vi "Move.vi"(6 "Cost":i32, 8 "Hallway Index":i32, 9 "Column Index":i32, 10 "Column":string, 11 "Data In":T1) -> (3 "Data Out":T1)   [LabVIEW 2020]
uses:
  Data.ctl
  <userlib>/_OpenG.lib/array/array.llb/Index 1D Array Elements (String)__ogtk.vi
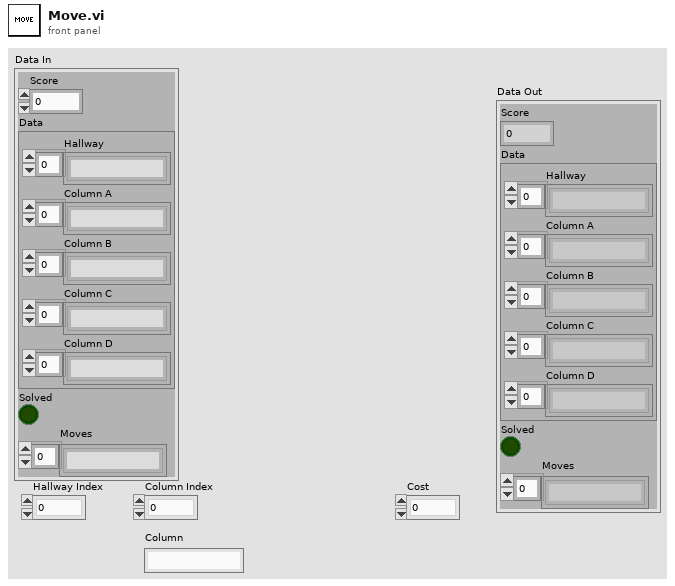
[diagram p1: front panel]
types:
  T1 = typedef "Data.ctl" = cluster{"Score":i64, "Data":cluster{"Hallway":string[], "Column A":string[], "Column B":string[], "Column C":string[], "Column D":string[]}, "Solved":bool, "Moves":string[]}
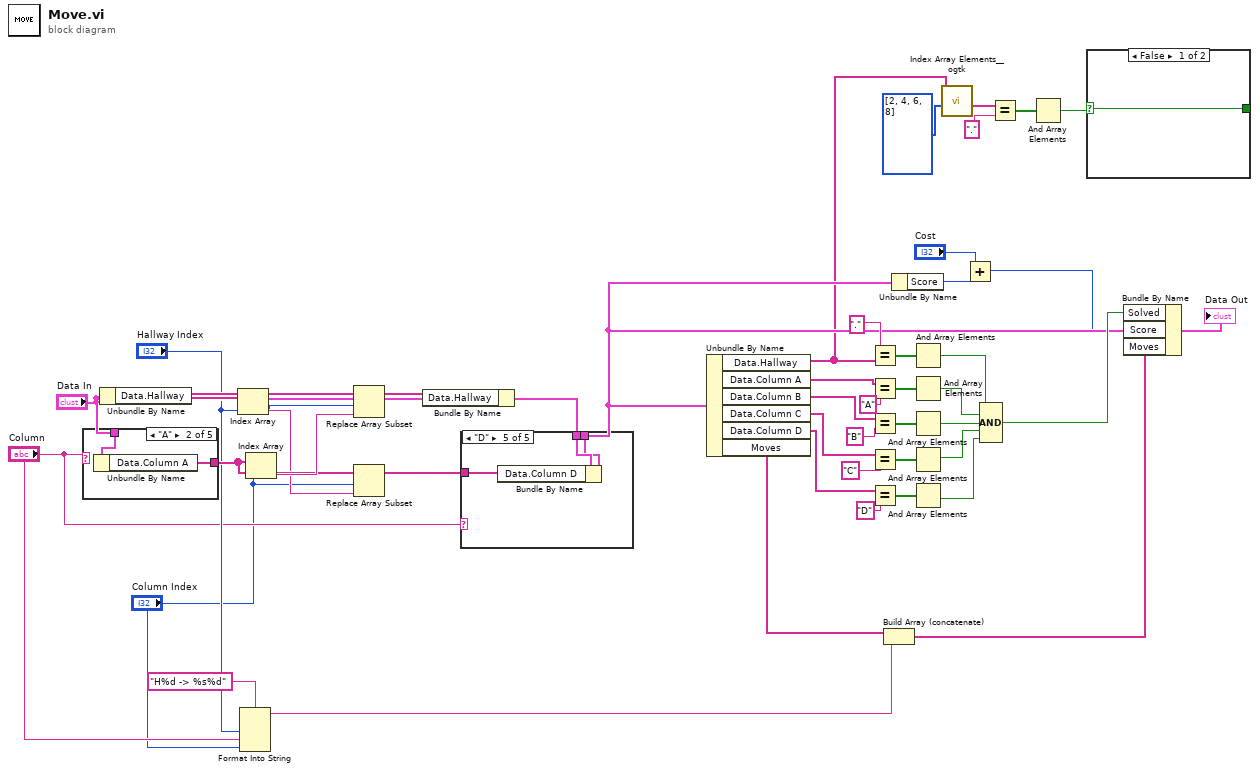
[diagram p0: block diagram]
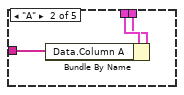
[diagram p4: hidden frame]
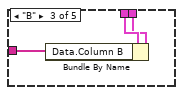
[diagram p5: hidden frame]
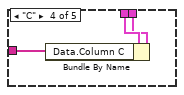
[diagram p6: hidden frame]
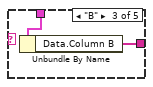
[diagram p8: hidden frame]
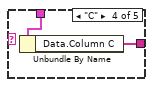
[diagram p9: hidden frame]
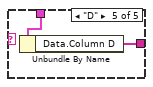
[diagram p10: hidden frame]
diagram:
  n1 = case shown="\"A\"" "Column" {
    tunnel: "Data In" -> [_ w48 w50 w52 w54]
    tunnel: [_ w47 w49 w51 w53] -> w44
    frame Default {
    }
    frame "A" {
      n2 = Unbundle By Name(w48) -> ("Data.Column A"=w47:string[])
    }
    frame "B" {
      n3 = Unbundle By Name(w50) -> ("Data.Column B"=w49:string[])
    }
    frame "C" {
      n4 = Unbundle By Name(w52) -> ("Data.Column C"=w51:string[])
    }
    frame "D" {
      n5 = Unbundle By Name(w54) -> ("Data.Column D"=w53:string[])
    }
  }
  n6 = Unbundle By Name("Data In") -> ("Data.Hallway"=w46:string[])
  n7 = Index Array(array=w46, index="Hallway Index") -> (element=w43:string)
  n8 = Format Into String(format string="H%d -> %s%d", "Hallway Index", "Column", "Column Index") -> (resulting string=w2:string)  [unwired: 2 in, 1 out]
  n9 = Index Array(array=w44, index="Column Index") -> (element=w45:string)
  n10 = Replace Array Subset(array=w46, new element=w45, index="Hallway Index") -> (w42:string[])
  n11 = Replace Array Subset(array=w44, new element=w43, index="Column Index") -> (w41:string[])
  n12 = Bundle By Name(cluster="Data In", "Data.Hallway"=w42) -> (w40:T1)
  n13 = case shown="\"D\"" "Column" {
    tunnel: w41 -> [_ w56 w59 w62 w65]
    tunnel: w40 -> [w55 w58 w61 w64 w67]
    tunnel: [w55 w57 w60 w63 w66] -> w18
    frame Default {
    }
    frame "A" {
      n14 = Bundle By Name(cluster=w58, "Data.Column A"=w56) -> (w57:T1)
    }
    frame "B" {
      n15 = Bundle By Name(cluster=w61, "Data.Column B"=w59) -> (w60:T1)
    }
    frame "C" {
      n16 = Bundle By Name(cluster=w64, "Data.Column C"=w62) -> (w63:T1)
    }
    frame "D" {
      n17 = Bundle By Name(cluster=w67, "Data.Column D"=w65) -> (w66:T1)
    }
  }
  n18 = Unbundle By Name(w18) -> ("Data.Hallway"=w14:string[], "Data.Column A"=w33:string[], "Data.Column B"=w32:string[], "Data.Column C"=w31:string[], "Data.Column D"=w4:string[], "Moves"=w3:string[])
  n19 = Equal?(x=".", y=w14) -> (x = y?=w38:bool[])
  n20 = Equal?(x=w33, y="A") -> (x = y?=w36:bool[])
  n21 = Equal?(x=w32, y="B") -> (x = y?=w37:bool[])
  n22 = Equal?(x=w31, y="C") -> (x = y?=w35:bool[])
  n23 = Equal?(x=w4, y="D") -> (x = y?=w34:bool[])
  n24 = Build Array (concatenate)(w3, w2) -> (w1:string[])
  n25 = Unbundle By Name(w18) -> ("Score"=w17:i64)
  n26 = And Array Elements(Boolean array=w38) -> (logical AND=w26:bool)
  n27 = And Array Elements(Boolean array=w36) -> (logical AND=w25:bool)
  n28 = And Array Elements(Boolean array=w37) -> (logical AND=w24:bool)
  n29 = And Array Elements(Boolean array=w35) -> (logical AND=w23:bool)
  n30 = And Array Elements(Boolean array=w34) -> (logical AND=w22:bool)
  n31 = call-poly <userlib>:"Index Array Elements__ogtk.vi"("indices"=i32[] [2, 4, 6, 8], "array"=w14) -> ("elements"=w11:string[])  [unwired: 9 in]
  n32 = Add(x="Cost", y=w17) -> (x+y=w15:i64)
  n33 = Compound Arithmetic op=AND(w26, w25, w24, w23, w22) -> (w20:bool)
  n34 = Equal?(x=w11, y=".") -> (x = y?=w12:bool[])
  n35 = And Array Elements(Boolean array=w12) -> (logical AND=w9:bool)
  n36 = case shown="False" w9 {
    selector: w9 -> [w68 w69]
    tunnel: [w68 w69] -> _
    frame False {
    }
    frame True {
    }
  }
  n37 = Bundle By Name(cluster=w18, "Solved"=w20, "Score"=w15, "Moves"=w1) -> (→"Data Out":T1)
